vi "modbus slave new.vi"() -> ()   [LabVIEW 2016]
uses:
  <vilib>/NI/Modbus Library/API/Wrapper/Create TCP Slave.vi
  <vilib>/NI/Modbus Library/API/slave/Modbus Slave.lvclass
  <vilib>/NI/Modbus Library/API/Wrapper/API Main.lvlib
  <vilib>/ptbypt/NI_PtbyPt.lvlib
  <vilib>/Utility/config.llb/NI_LVConfig.lvlib
panel:
  out "读取register values 2":u16[](array[numeric])
  out "status":bool
  in  "写入registers to write":u16[](array[numeric])
  out "读取register values":u16[](array[numeric])
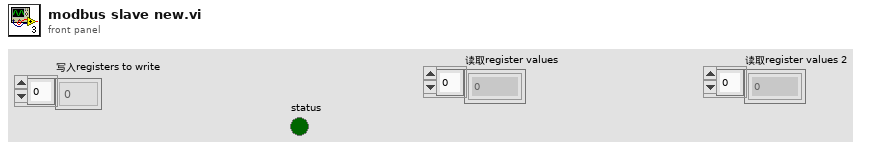
[diagram p1: front panel]
types:
  T1 = enum16{"启动整机", "停止整机", "标样核查", "加标回收", "平行样测试", "零点核查", "跨度核查", "校零", "校标"}
  T2 = cluster{"status":bool, "代码":u16, "source":string}
  T3 = cluster{"COD浓度（mg/L)":dbl, "水样启动时间":timestamp, "加标回收启动时间":timestamp, "CODMn工作状态":enum16{"空闲", "水样测试", "标样核查", "零点核查", "跨度核查", "空白测试", "平行样测试", "加标回收", "空白校准", "标样校准", "初始化（清洗）"}, "多列列表框":i32}
  T4 = cluster{"系统时间":timestamp, "工作状态":u16, "测量模式":enum16{"待机", "连续模式", "周期模式", "定点模式", "受控模式", "手动模式"}, "告警代码":u16, "故障代码":u16, "日志代码":u16, "软件版本":u16, "F0":sgl, "F1":sgl, "F2":sgl, "F3":sgl, "T":sgl, "H":sgl, "id":u16, "flowid":u16, "量程":u16, "总磷控温温度1":sgl, "营养盐控温温度2":sgl, "ADC":sgl}
  T5 = enum16{"空闲", "水样测试", "标样核查", "零点核查", "跨度核查", "空白测试", "平行样测试", "加标回收", "空白校准", "标样校准", "初始化（清洗）"}
  T6 = typedef "NI_LVConfig.lvlib/Config Data RefNum.ctl" = refnum<k1>
  T7 = enum16{"", "CODMn", "PH", "氨氮", "总氮", "总磷", "CODCr", "电导率", "水温", "溶解氧", "浊度", "叶绿素", "藻密度", "ORP"}
  T8 = enum16{"i13001", "i13002", "i13003", "i13004", "i13005", "i13006", "i13007", "i13008", "i13009", "i13010", "i13011", "i13012", "i13013", "i13014", "i13015", "i13016", "i13017", "i13101", "i13102", "i13103", "i13104", "i13105", "i13106", "i13107", "i13108", "i13109", "i13110"}
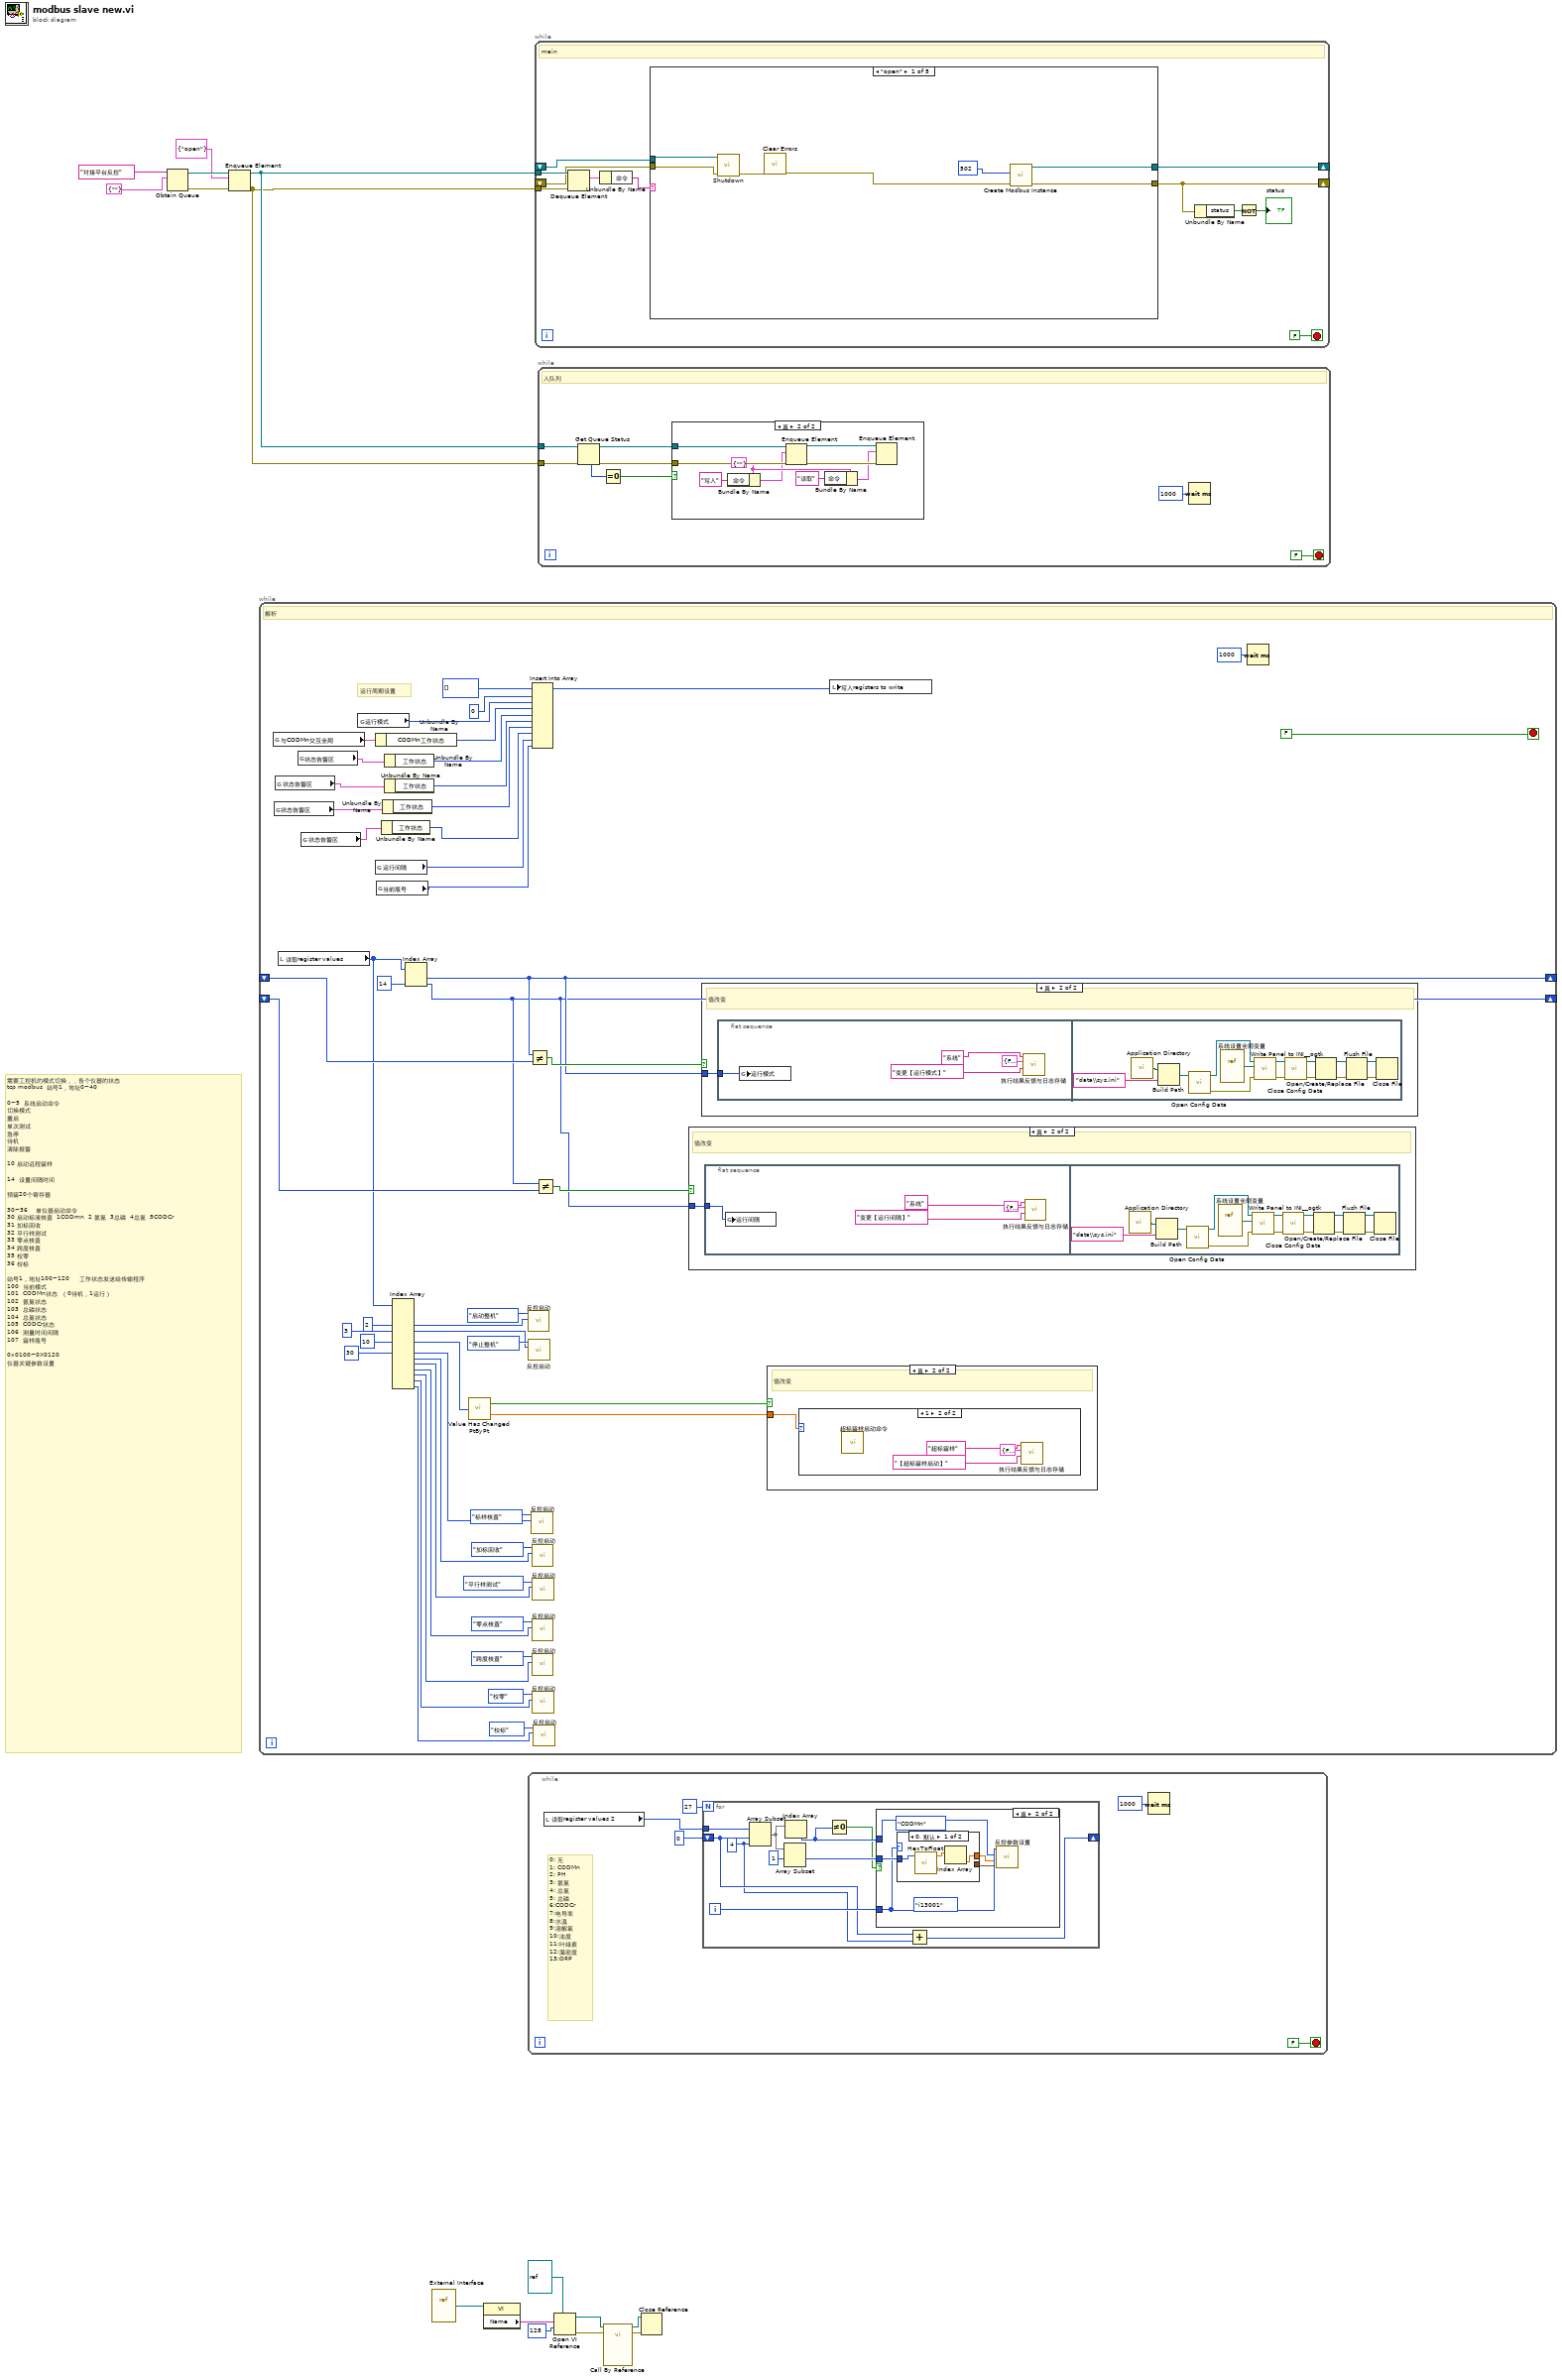
[diagram p0: block diagram]
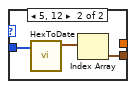
[diagram p3: hidden frame]
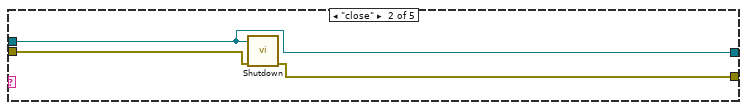
[diagram p9: hidden frame]
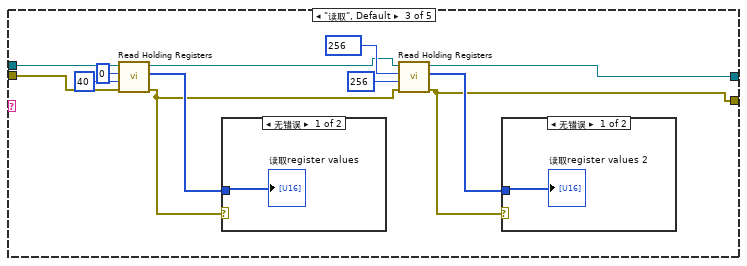
[diagram p10: hidden frame]
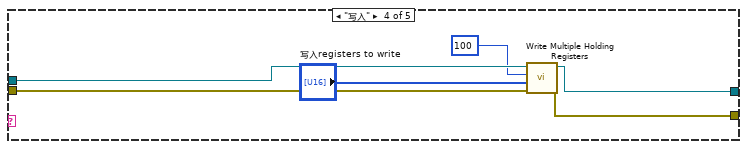
[diagram p13: hidden frame]
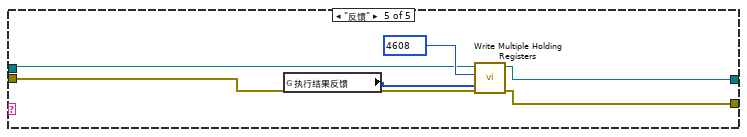
[diagram p14: hidden frame]
diagram:
  # "需要工控机的模式切换，，各个仪器的状态\ntcp modbus  站号1，地址0~40\n\n0~5  系统启动命令\n切换模式\n重启\n单次测试\n急停\n待机\n清除报警\n\n10 启动远程留样\n\n14  设置间隔时间\n\n预留20个寄存器\n\n30~36    单仪器启动命令\n30 启动标液核查  1CODmn  2 氨氮  3总磷  4总氮  5CODCr\n31 加标回收\n32 平行样测试\n33 零点核查\n34 跨度核查\n35 校零\n36 校标\n\n站号1，地址100~120     工作状态发送给传输程序\n100  当前模式\n101  CODMn状态  （0待机，1运行）\n102  氨氮状态\n103  总磷状态\n104  总氮状态\n105  CODCr状态\n106  测量时间间隔\n107  留样瓶号\n\n0x0100~0X0120\n仪器关键参数设置"
  n1 = Obtain Queue(name (unnamed)="对接平台反控" ("名称（未命名）"), element data type=cluster{"命令":string} {"命令"=""}) -> (queue out=w13:refnum<queue>, error out=w12:errorcluster)  [unwired: 3 in, 1 out]
  n2 = Enqueue Element(queue=w13, element=cluster{"命令":string} {"命令"="open"} ("元素"), error in (no error)=w12) -> (queue out=w10:refnum<queue>, error out=w9:errorcluster)  [unwired: 1 in, 1 out]
  n3 = while {
    shift-right: [w53] -> _
    shift-left: _ -> [w55]
    shift-right: [w50] -> _
    shift-left: _ -> [w52]
    stop <- FALSE stop-if-true
    # "运行周期设置"
    # "解析"
    n4 = global read "modbus slave全局.vi" "与CODMn交互全局"() -> (w22:T3)
    n5 = global read "VAR总磷总氮全局变量.vi" "状态告警区"() -> (w16:T4)
    n6 = global read "VAR总磷总氮全局变量.vi" "状态告警区"() -> (w17:T4)
    n7 = local read "读取register values"() -> (w45:u16[])
    n8 = global read "VAR总磷总氮全局变量.vi" "状态告警区"() -> (w20:T4)
    n9 = global read "VAR总磷总氮全局变量.vi" "状态告警区"() -> (w19:T4)
    n10 = global read "系统设置全局变量.vi" "运行模式"() -> (w63:enum16{"维护模式", "常规模式", "应急模式", "质控模式"})
    n11 = Unbundle By Name(w22) -> ("CODMn工作状态"=w21:T5)
    n12 = global read "系统设置全局变量.vi" "运行间隔"() -> (w58:i16)
    n13 = global read "外部交互全局.vi" "当前瓶号"() -> (w23:u16)
    n14 = Unbundle By Name(w19) -> ("工作状态"=w18:u16)
    n15 = Unbundle By Name(w16) -> ("工作状态"=w59:u16)
    n16 = Unbundle By Name(w20) -> ("工作状态"=w61:u16)
    n17 = Unbundle By Name(w17) -> ("工作状态"=w60:u16)
    n18 = Index Array(array=w45, index #3=2 ("索引"), index #4=3 ("索引"), index #6=10 ("索引"), index #8=30 ("索引")) -> (element #3=w44:u16, element #4=w41:u16, element #6=w38:u16, element #8=w36:u16, element #9=w30:u16, element #10=w29:u16, element #11=w28:u16, element #12=w26:u16, element #13=w25:u16, element #14=w24:u16)  [unwired: 10 in, 4 out]
    n19 = Index Array(array=w45, index #2=14 ("索引")) -> (element #1=w53:u16, element #2=w50:u16)  [unwired: 1 in]
    n20 = call <vilib>:"Value Has Changed PtByPt.vi"("input data point"=w38) -> ("has changed"=w40:bool, "output data point"=w39:dbl)  [unwired: 1 in]
    n21 = call "反控启动.vi"("启动参数"=w44, "启动类型"=T1."启动整机") -> ()  [unwired: 10 in]
    n22 = call "反控启动.vi"("启动参数"=w41, "启动类型"=T1."停止整机") -> ()  [unwired: 10 in]
    n23 = Not Equal?(x=w53, y=w55) -> (x != y?=w54:bool)
    n24 = call "反控启动.vi"("启动参数"=w36, "启动类型"=T1."标样核查") -> ()  [unwired: 10 in]
    n25 = Insert Into Array(array=u16[] [] ("values to write"), index=0 ("索引"), new element #1=w63, new element #2=w21, new element #3=w61, new element #4=w60, new element #5=w59, new element #6=w18, new element #7=w58, new element #8=w23) -> (w57:u16[])
    n26 = call "反控启动.vi"("启动参数"=w30, "启动类型"=T1."加标回收") -> ()  [unwired: 10 in]
    n27 = call "反控启动.vi"("启动参数"=w28, "启动类型"=T1."零点核查") -> ()  [unwired: 10 in]
    n28 = call "反控启动.vi"("启动参数"=w26, "启动类型"=T1."跨度核查") -> ()  [unwired: 10 in]
    n29 = call "反控启动.vi"("启动参数"=w29, "启动类型"=T1."平行样测试") -> ()  [unwired: 10 in]
    n30 = call "反控启动.vi"("启动参数"=w25, "启动类型"=T1."校零") -> ()  [unwired: 10 in]
    n31 = call "反控启动.vi"("启动参数"=w24, "启动类型"=T1."校标") -> ()  [unwired: 10 in]
    n32 = Not Equal?(x=w50, y=w52) -> (x != y?=w51:bool)
    n33 = case shown="真" w51 {
      tunnel: w50 -> [_ w71]
      frame False {
      }
      frame True {
        # "值改变"
        n34 = flat-sequence {
          tunnel: w71 -> [w75]
          frame #0 {
            n35 = global write "系统设置全局变量.vi" "运行间隔"(w75) -> ()
            n36 = call "执行结果反馈与日志存储.vi"("日志信息"="变更【运行间隔】", "error out"=T2 {"status"=FALSE, "代码"=1, "source"=""}, "设备"="系统") -> ()  [unwired: 9 in]
          }
          frame #1 {
            n37 = call <vilib>:"Application Directory.vi"() -> ("Application Directory"=w89:path)
            n38 = Build Path(base path=w89, name or relative path="data\\sys.ini" ("名称或相对路径")) -> (appended path=w87:path)
            n39 = call <vilib>:"Open Config Data.vi"("configuration file path"=w87) -> ("error out"=w83:errorcluster, "refnum"=w86:T6)  [unwired: 8 in, 1 out]
            n40 = vi-ref "系统设置全局变量.vi"() -> (w85:refnum<vi>)
            n41 = call <userlib>:"Write Panel to INI__ogtk.vi"("error in (no error)"=w83, "VI ref"=w85, "refnum"=w86) -> ("error out"=w82:errorcluster, "refnum out"=w84:T6)  [unwired: 7 in]
            n42 = call <vilib>:"Close Config Data.vi"("error in (no error)"=w82, "refnum"=w84) -> ("error out"=w77:errorcluster, "file path"=w76:path)  [unwired: 8 in]
            n43 = Open/Create/Replace File(file path (use dialog)=w76, error in=w77) -> (refnum out=w80:refnum<file>, error out=w81:errorcluster)  [unwired: 4 in, 1 out]
            n44 = Flush File(refnum=w80, error in=w81) -> (refnum out=w79:refnum<file>, error out=w78:errorcluster)
            n45 = Close File(refnum=w79, error in=w78) -> ()  [unwired: 2 out]
          }
        }
      }
    }
    n46 = case shown="真" w54 {
      tunnel: w53 -> [_ w90]
      frame False {
      }
      frame True {
        # "值改变"
        n47 = flat-sequence {
          tunnel: w90 -> [w94]
          frame #0 {
            n48 = global write "系统设置全局变量.vi" "运行模式"(w94) -> ()
            n49 = call "执行结果反馈与日志存储.vi"("日志信息"="变更【运行模式】", "error out"=T2 {"status"=FALSE, "代码"=1, "source"=""}, "设备"="系统") -> ()  [unwired: 9 in]
          }
          frame #1 {
            n50 = call <vilib>:"Application Directory.vi"() -> ("Application Directory"=w108:path)
            n51 = Build Path(base path=w108, name or relative path="data\\sys.ini" ("名称或相对路径")) -> (appended path=w106:path)
            n52 = call <vilib>:"Open Config Data.vi"("configuration file path"=w106) -> ("error out"=w102:errorcluster, "refnum"=w105:T6)  [unwired: 8 in, 1 out]
            n53 = vi-ref "系统设置全局变量.vi"() -> (w104:refnum<vi>)
            n54 = call <userlib>:"Write Panel to INI__ogtk.vi"("error in (no error)"=w102, "VI ref"=w104, "refnum"=w105) -> ("error out"=w101:errorcluster, "refnum out"=w103:T6)  [unwired: 7 in]
            n55 = call <vilib>:"Close Config Data.vi"("error in (no error)"=w101, "refnum"=w103) -> ("error out"=w96:errorcluster, "file path"=w95:path)  [unwired: 8 in]
            n56 = Open/Create/Replace File(file path (use dialog)=w95, error in=w96) -> (refnum out=w99:refnum<file>, error out=w100:errorcluster)  [unwired: 4 in, 1 out]
            n57 = Flush File(refnum=w99, error in=w100) -> (refnum out=w98:refnum<file>, error out=w97:errorcluster)
            n58 = Close File(refnum=w98, error in=w97) -> ()  [unwired: 2 out]
          }
        }
      }
    }
    n59 = case shown="真" w40 {
      tunnel: w39 -> [_ w67]
      frame False {
      }
      frame True {
        # "值改变"
        n60 = case shown="1" w67 {
          frame 0, Default {
          }
          frame 1 {
            n61 = call "超标留样启动命令.vi"() -> ()  [unwired: 12 in]
            n62 = call "执行结果反馈与日志存储.vi"("日志信息"="【超标留样启动】", "error out"=T2 {"status"=FALSE, "代码"=1, "source"=""}, "设备"="超标留样") -> ()  [unwired: 9 in]
          }
        }
      }
    }
    n63 = local write "写入registers to write"(w57) -> ()
    n64 = Wait (ms)(milliseconds to wait=u32 1000 ("等待时间（毫秒）")) -> ()  [unwired: 1 out]
  }
  n65 = vi-ref "External Interface.vi"() -> (w8:refnum<vi>)
  n66 = property class="VI"(reference=w8) -> ("Name"=w7:string)  [unwired: 1 in, 2 out]
  n67 = while {
    stop <- FALSE stop-if-true
    # "0: 无\n1: CODMn\n2: PH\n3: 氨氮\n4: 总氮\n5: 总磷\n6:CODCr\n7:电导率\n8:水温\n9:溶解氧\n10:浊度\n11:叶绿素\n12:藻密度\n13:ORP"
    n68 = local read "读取register values 2"() -> (w111:u16[])
    n69 = for {
      N: 27 -> [_]
      tunnel: w111 -> [w123]
      shift-right: [w114] -> _
      shift-left: 0 ("索引") -> [w116]
      i -> [w119]
      w115 = 4 ("长度")
      n70 = Array Subset(array=w123, index=w116, length=w115) -> (w122:u16[])
      n71 = Array Subset(array=w122, index=1 ("索引")) -> (w120:u16[])  [unwired: 1 in]
      n72 = Index Array(array=w122) -> (element=w118:u16)  [unwired: 1 in]
      n73 = Not Equal To 0?(x=w118) -> (x != 0?=w117:bool)
      n74 = case shown="真" w117 {
        tunnel: w120 -> [_ w128]
        tunnel: w119 -> [_ w127]
        tunnel: w118 -> [_ w126]
        frame False {
        }
        frame True {
          (unwired) T7."CODMn"
          (unwired) T8."i13001" ("设置类型")
          n75 = case shown="0, 默认" w127 {
            tunnel: w128 -> [w130 w133]
            tunnel: [_ w134] -> w124
            tunnel: [w131 _] -> w125
            frame 0, Default {
              n76 = call "HexToFloat.vi"("数组"=w130) -> ("FLOAT"=w129:sgl[])  [unwired: 10 in]
              n77 = Index Array(array=w129) -> (element=w131:sgl)  [unwired: 1 in]
            }
            frame 5, 12 {
              n78 = call "HexToDate.vi"("数组"=w133) -> ("DATE"=w132:timestamp[])  [unwired: 10 in]
              n79 = Index Array(array=w132) -> (element=w134:timestamp)  [unwired: 1 in]
            }
          }
          n80 = call "反控参数设置.vi"("value time"=w124, "value float"=w125, "设置参数"=w126, "设置类型"=w127) -> ()  [unwired: 8 in]
        }
      }
      n81 = Add(x=w116, y=w115) -> (x+y=w114:i32)
    }
    n82 = Wait (ms)(milliseconds to wait=u32 1000 ("等待时间（毫秒）")) -> ()  [unwired: 1 out]
  }
  n83 = while {
    tunnel: w10 -> [w145]
    tunnel: w9 -> [w144]
    shift-right: [w141] -> _
    shift-left: _ -> [w140]
    shift-right: [w135] -> _
    shift-left: _ -> [w139]
    stop <- FALSE stop-if-true
    # "main"
    n84 = Dequeue Element(queue=w145, error in (no error)=w144) -> (element=w143:cluster{"命令":string})  [unwired: 1 in, 3 out]
    n85 = Unbundle By Name(w143) -> ("命令"=w142:string)
    n86 = case shown="\"open\"" w142 {
      tunnel: [w150 w153 w157 w171 w178] -> w141
      tunnel: [w151 w154 w156 w170 w177] -> w135
      tunnel: w140 -> [w149 w153 w167 w175 w180]
      tunnel: w139 -> [w148 w155 w166 w174 w179]
      frame "open" {
        n87 = call-dynamic "Shutdown.vi"("error in"=w148, "Modbus slave in"=w149) -> ("error out"=w147:errorcluster)  [unwired: 9 in]
        n88 = call <vilib>:"Clear Errors.vi"("error in (no error)"=w147) -> ("error out"=w146:errorcluster)  [unwired: 5 in, 1 out]
        n89 = call-poly <vilib>:"Create Modbus Instance.vi"("error in"=w146, "port (502)"=u16 502) -> ("error out"=w151:errorcluster, "TCP slave instance"=w150:refnum<class "Modbus Slave.lvclass">)  [unwired: 8 in]
      }
      frame "close" {
        n90 = call-dynamic "Shutdown.vi"("error in"=w155, "Modbus slave in"=w153) -> ("error out"=w154:errorcluster)  [unwired: 9 in]
      }
      frame "读取", Default {
        n91 = call-dynamic "Read Holding Registers.vi"("error in"=w166, "number of inputs"=u16 40, "starting address"=u16 0, "Modbus slave in"=w167) -> ("error out"=w158:errorcluster, "register values"=w163:u16[], "Modbus slave out"=w159:refnum<class "Modbus Slave.lvclass">)  [unwired: 5 in]
        n92 = case shown="无错误" w158 {
          tunnel: w163 -> [w169 _]
          frame No Error {
            "读取register values" <- w169
          }
          frame Error {
          }
        }
        n93 = call-dynamic "Read Holding Registers.vi"("error in"=w158, "number of inputs"=u16 256, "starting address"=u16 256, "Modbus slave in"=w159) -> ("error out"=w156:errorcluster, "register values"=w162:u16[], "Modbus slave out"=w157:refnum<class "Modbus Slave.lvclass">)  [unwired: 5 in]
        n94 = case shown="无错误" w156 {
          tunnel: w162 -> [w168 _]
          frame No Error {
            "读取register values 2" <- w168
          }
          frame Error {
          }
        }
      }
      frame "写入" {
        n95 = call-dynamic "Write Multiple Holding Registers.vi"("error in"=w174, "registers to write"="写入registers to write", "starting address"=u16 100, "Modbus slave in"=w175) -> ("error out"=w170:errorcluster, "Modbus slave out"=w171:refnum<class "Modbus Slave.lvclass">)  [unwired: 6 in]
      }
      frame "反馈" {
        n96 = global read "modbus slave全局.vi" "执行结果反馈"() -> (w176:u16[])
        n97 = call-dynamic "Write Multiple Holding Registers.vi"("error in"=w179, "registers to write"=w176, "starting address"=u16 4608, "Modbus slave in"=w180) -> ("error out"=w177:errorcluster, "Modbus slave out"=w178:refnum<class "Modbus Slave.lvclass">)  [unwired: 6 in]
      }
    }
    n98 = Unbundle By Name(w135) -> ("status"=w137:bool)
    n99 = Not(x=w137) -> (.not. x?=→"status":bool)
  }
  n100 = while {
    tunnel: w10 -> [w189]
    tunnel: w9 -> [w187]
    stop <- FALSE stop-if-true
    # "入队列"
    n101 = Get Queue Status(queue=w189, error in (no error)=w187) -> (queue out=w188:refnum<queue>, error out=w186:errorcluster, # elements in queue=w185:i32)  [unwired: 1 in, 5 out]
    n102 = Equal To 0?(x=w185) -> (x = 0?=w184:bool)
    n103 = case shown="真" w184 {
      tunnel: w188 -> [_ w198]
      tunnel: w186 -> [_ w197]
      frame False {
      }
      frame True {
        w193 = cluster{"命令":string} {"命令"=""} ("元素")
        n104 = Bundle By Name(cluster=w193, "命令"="写入") -> (w192:cluster{"命令":string})
        n105 = Enqueue Element(queue=w198, element=w192, error in (no error)=w197) -> (queue out=w196:refnum<queue>, error out=w195:errorcluster)  [unwired: 1 in, 1 out]
        n106 = Bundle By Name(cluster=w193, "命令"="读取") -> (w190:cluster{"命令":string})
        n107 = Enqueue Element(queue=w196, element=w190, error in (no error)=w195) -> ()  [unwired: 1 in, 3 out]
      }
    }
    n108 = Wait (ms)(milliseconds to wait=u32 1000 ("等待时间（毫秒）")) -> ()  [unwired: 1 out]
  }
  n109 = Open VI Reference(type specifier VI Refnum (for type only)=refnum<vi> refnum, vi path=w7, options=128 ("选项")) -> (vi reference=w5:refnum<vi>, error out=w3:errorcluster)  [unwired: 3 in]
  n110 = call-by-ref "?"(reference=w5, error in=w3) -> (reference out=w1:refnum<vi>, error out=w2:errorcluster)  [unwired: 12 in]
  n111 = Close Reference(reference=w1, error in (no error)=w2) -> ()  [unwired: 1 out]
